vi "Process.vi"(8 "error in (no error)":errorcluster, 10 "Pound in":refnum<class "Pound.lvclass">, 11 "Qbus in":refnum<class "Qbus.lvclass">) -> (0 "error out":errorcluster)   [LabVIEW 2017, in "ServerComm.lvlib"]
doc: "Handles communication between the device and NI InsightCM Server."
uses:
  <vilib>/addons/InsightCM/Devices/Shared/Common/ServerComm/ServerComm.lvlib
  <vilib>/addons/Qbus/Qbus.lvclass
  <vilib>/NI/Software Watchdog/Pound/Pound.lvclass
  <vilib>/addons/InsightCM/Devices/Shared/Common/ServerComm/controls/config.ctl
  <vilib>/addons/InsightCM/MessageBus/TcpApi/controls/TcpMessageReference.ctl
  <vilib>/addons/InsightCM/MessageBus/Base/controls/ConnectionInfo.ctl
  <vilib>/addons/InsightCM/SRP/controls/DVR_data.ctl
  <vilib>/addons/InsightCM/SRP/controls/data.ctl
  <vilib>/addons/InsightCM/Devices/Shared/Common/ServerComm/controls/ConnectedStatusDvr.ctl
  <vilib>/addons/InsightCM/Devices/Shared/Common/ServerComm/controls/ConnectionStatus.ctl
  <vilib>/addons/InsightCM/Devices/Shared/Common/ServerComm/controls/DataSendStatus.ctl
  <vilib>/addons/InsightCM/Devices/Shared/Common/ServerComm/controls/DataSendMode.ctl
  <vilib>/addons/InsightCM/Devices/Shared/Common/ServerComm/controls/ReconnectData.ctl
  <vilib>/addons/InsightCM/Devices/Shared/Common/ServerComm/controls/ProvisioningVersionInfo.ctl
  <vilib>/addons/InsightCM/MessageBus/MessageLibrary/Authentication/controls/AuthSrpVerificationRequestBody.ctl
  <vilib>/addons/InsightCM/Devices/Shared/Common/ServerComm/controls/TimerFunction.ctl
  <vilib>/addons/InsightCM/MessageBus/MessageLibrary/Transceiver/controls/TransAuthorizePortRequestBody.ctl
  <vilib>/addons/InsightCM/MessageBus/MessageLibrary/Device/controls/DeviceInvalidConfigurationBroadcastBody.ctl
  <vilib>/addons/InsightCM/MessageBus/Base/controls/IRoutingSource.ctl
  <vilib>/addons/InsightCM/Devices/Shared/Common/ServerComm/controls/DataSendBody.ctl
  <vilib>/addons/InsightCM/MessageBus/MessageLibrary/Authentication/controls/AuthSrpInitiationRequestBody.ctl
  <vilib>/addons/InsightCM/MessageBus/MessageLibrary/DataStorage/controls/DataStorageOpenEventRequestBody.ctl
  <vilib>/addons/InsightCM/MessageBus/Base/controls/KeyValuePair.ctl
  <vilib>/addons/TraceLogger/TraceLogger.lvlib
  <vilib>/NI/Software Watchdog/Watchdog/Watchdog.lvclass
  <vilib>/addons/InsightCM/SRP/SRP.lvlib
  <vilib>/addons/InsightCM/Utilities/GlobalConfiguration/GlobalConfiguration.lvlib
  <vilib>/addons/InsightCM/Devices/Shared/Common/TracePointSynchronizer/TracePointSynchronizer.lvlib
  <vilib>/addons/InsightCM/Devices/Shared/Common/USBDrive/USBDrive.lvlib
  <vilib>/addons/SystemInfoProcess/SystemInfoProcess.lvlib
  <vilib>/addons/InsightCM/Utilities/PropertyHelpers/PropertyHelpers.lvlib
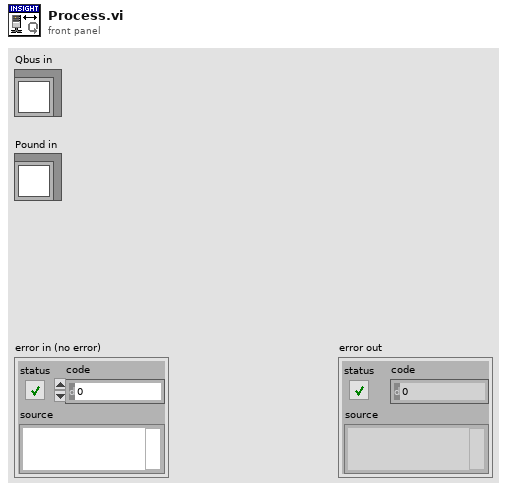
[diagram p1: front panel]
types:
  T1 = typedef "ServerComm.lvlib/config.ctl" = cluster{"tcp":T2, "ConnInfo":T3, "SRP":T4, "connected":T5, "DataSend":T6, "Reconnect":T8, "ProvVersionInfo":T9}
  T2 = typedef "TcpMessageReference.ctl" = refnum<data-value>
  T3 = typedef "ConnectionInfo.ctl" = cluster{"ClientName":string, "TransceiverHost":string, "TransceiverPort":u16, "Password":string}
  T4 = typedef "SRP.lvlib/DVR_data.ctl" = refnum<data-value>
  T5 = typedef "ServerComm.lvlib/ConnectedStatusDvr.ctl" = refnum<data-value>
  T6 = typedef "ServerComm.lvlib/DataSendStatus.ctl" = cluster{"SendFileMode":T7, "data":variant, "InProgress":bool}
  T7 = typedef "ServerComm.lvlib/DataSendMode.ctl" = enum16{"File", "InMemoryFile", "Stream", "StreamFileBlock", "ByteArray", "NoOp", "UnknownData"}
  T8 = typedef "ServerComm.lvlib/ReconnectData.ctl" = cluster{"ReconnectInterval":dbl, "BaseReconnectInterval":dbl, "AuthAttempts":i32, "MaxAttempts":i32}
  T9 = typedef "ServerComm.lvlib/ProvisioningVersionInfo.ctl" = cluster{"ConfigurationVersion":string, "ApplicationVersion":string, "ApplicationType":string}
  T10 = typedef "SectionKeyValues.ctl" = cluster{"Section":string, "KeyValues":T11[]}
  T11 = typedef "KeyValuePair.ctl" = cluster{"Key":string, "Value":string}
  T12 = typedef "ServerComm.lvlib/ConnectionStatus.ctl" = enum16{"Offline", "NotAuthorized", "Online"}
  T13 = typedef "ServerComm.lvlib/TimerFunction.ctl" = enum16{"Start", "Stop", "Reset"}
  T14 = typedef "AuthSrpVerificationRequestBody.ctl" = cluster{"ClientName":string, "ClientHashM":u8[]}
  T15 = typedef "TransAuthorizePortRequestBody.ctl" = cluster{"DeviceName":string, "ConnectionId":string}
  T16 = typedef "DeviceInvalidConfigurationBroadcastBody.ctl" = cluster{"DeviceName":string, "Description":string}
  T17 = typedef "ServerComm.lvlib/DataSendBody.ctl" = cluster{"tcp reference":T2, "SendFileMode":T7, "data":variant, "IRoutingSource":T18, "ReplyTo":string}
  T18 = typedef "IRoutingSource.ctl" = cluster{"CorrelationId":string, "ReplyTo":string}
  T19 = typedef "AuthSrpInitiationRequestBody.ctl" = cluster{"ClientName":string, "PublicKeyA":u8[]}
  T20 = typedef "DataStorageOpenEventRequestBody.ctl" = cluster{"EventId":string, "Properties":T11[]}
  T21 = typedef "Message.ctl" = cluster{"Header":T22, "Body":u8[]}
  T22 = typedef "MessageHeader.ctl" = cluster{"MessageName":string, "Timestamp":i64, "CorrelationId":string, "ContentType":string, "RoutingKey":string, "Properties":T11[]}
  T23 = typedef "AuthSrpInitiationResponseBody.ctl" = cluster{"Salt":u8[], "PublicKeyB":u8[]}
  T24 = typedef "AuthSrpVerificationResponseBody.ctl" = cluster{"ServerHashM":u8[]}
  T25 = typedef "DeviceConnectionInfoUpdateRoutedMessageBody.ctl" = cluster{"IV":u8[], "ConnectionInfo":u8[]}
  T26 = typedef "DeviceConfigurationUpdateRoutedMessageBody.ctl" = cluster{"Config":T27}
  T27 = typedef "DeviceProvisioning.ctl" = cluster{"DeviceModel":T28}
  T28 = typedef "DeviceModel.ctl" = cluster{"Device":T29, "Channels":T38[], "Tags":T39[]}
  T29 = typedef "Device.ctl" = cluster{"Id":string, "Name":string, "DeviceType":string, "HardwareName":string, "IpAddress":string, "HardwareInfo":T11[], "ApplicationType":string, "ApplicationVersion":string, "ConfigurationVersion":string, "State":T30, "Properties":T11[], "DataGroups":T31[], "BurstModeTrigger":T32, "SensorGroups":T35[], "HasSensorGroups":bool, "Endpoints":T36[]}
  T30 = typedef "DeviceState.ctl" = cluster{"Disabled":bool}
  T31 = typedef "DataGroup.ctl" = cluster{"Name":string, "AssetNodeId":string}
  T32 = typedef "BurstModeTrigger.ctl" = cluster{"Trigger":T33, "SampleRate":string, "AcquisitionLength":string}
  T33 = typedef "Trigger.ctl" = cluster{"Type":string, "Expression":string, "Conditions":T34[]}
  T34 = typedef "Condition.ctl" = cluster{"Source":string, "Type":string, "Operator":string, "CompareTo":string, "DwellSeconds":dbl}
  T35 = typedef "DeviceSensorGroup.ctl" = cluster{"EquipId":string, "SensorGroupId":string}
  T36 = typedef "WirelessEndpoint.ctl" = cluster{"SerialNumber":string, "Properties":T11[], "Channels":T37[]}
  T37 = typedef "WirelessChannel.ctl" = cluster{"ChannelNumber":i32, "AssetId":string}
  T38 = typedef "Channel.ctl" = cluster{"Id":string, "DeviceId":string, "ChannelType":string, "HardwareKey":string, "HardwareChannel":string, "DataGroup":string, "Properties":T11[], "AssetNodeId":string}
  T39 = typedef "Tag.ctl" = cluster{"Id":string, "Path":string, "Name":string, "Datatype":string, "Props":T11[], "Keywords":string[]}
  T40 = typedef "DeviceSetNiAuthPasswordRequestBody.ctl" = cluster{"IV":u8[], "Password":u8[]}
  T41 = typedef "ServerComm.lvlib/UpdatePassword.ctl" = cluster{"Device Id":string, "Serial Number":string, "New Password":string}
  T42 = typedef "R2_Device.ctl" = cluster{"Id":string, "Name":string, "DeviceType":string, "HardwareName":string, "IpAddress":string, "HardwareInfo":T11[], "ApplicationType":string, "ApplicationVersion":string, "EquipmentIds":string[], "ConfigurationVersion":string, "State":T30, "Properties":T11[], "DataGroups":T43[], "BurstModeTrigger":T32, "SensorGroups":T35[], "Endpoints":T36[]}
  T43 = typedef "R2_DataGroup.ctl" = cluster{"Name":string, "OperatingStates":T44[], "Properties":T11[], "EquipmentIds":string[], "AssetNodeId":string}
  T44 = typedef "OperatingState.ctl" = cluster{"Name":string, "Properties":T11[], "Triggers":T33[]}
  T45 = typedef "PointValueMap.lvlib/PointMap.ctl" = refnum<data-value>
  T46 = typedef "SystemInfoProcess.lvlib/ImageMetadata.ctl" = cluster{"Title":string, "Description":string, "ID":string, "Version":string}
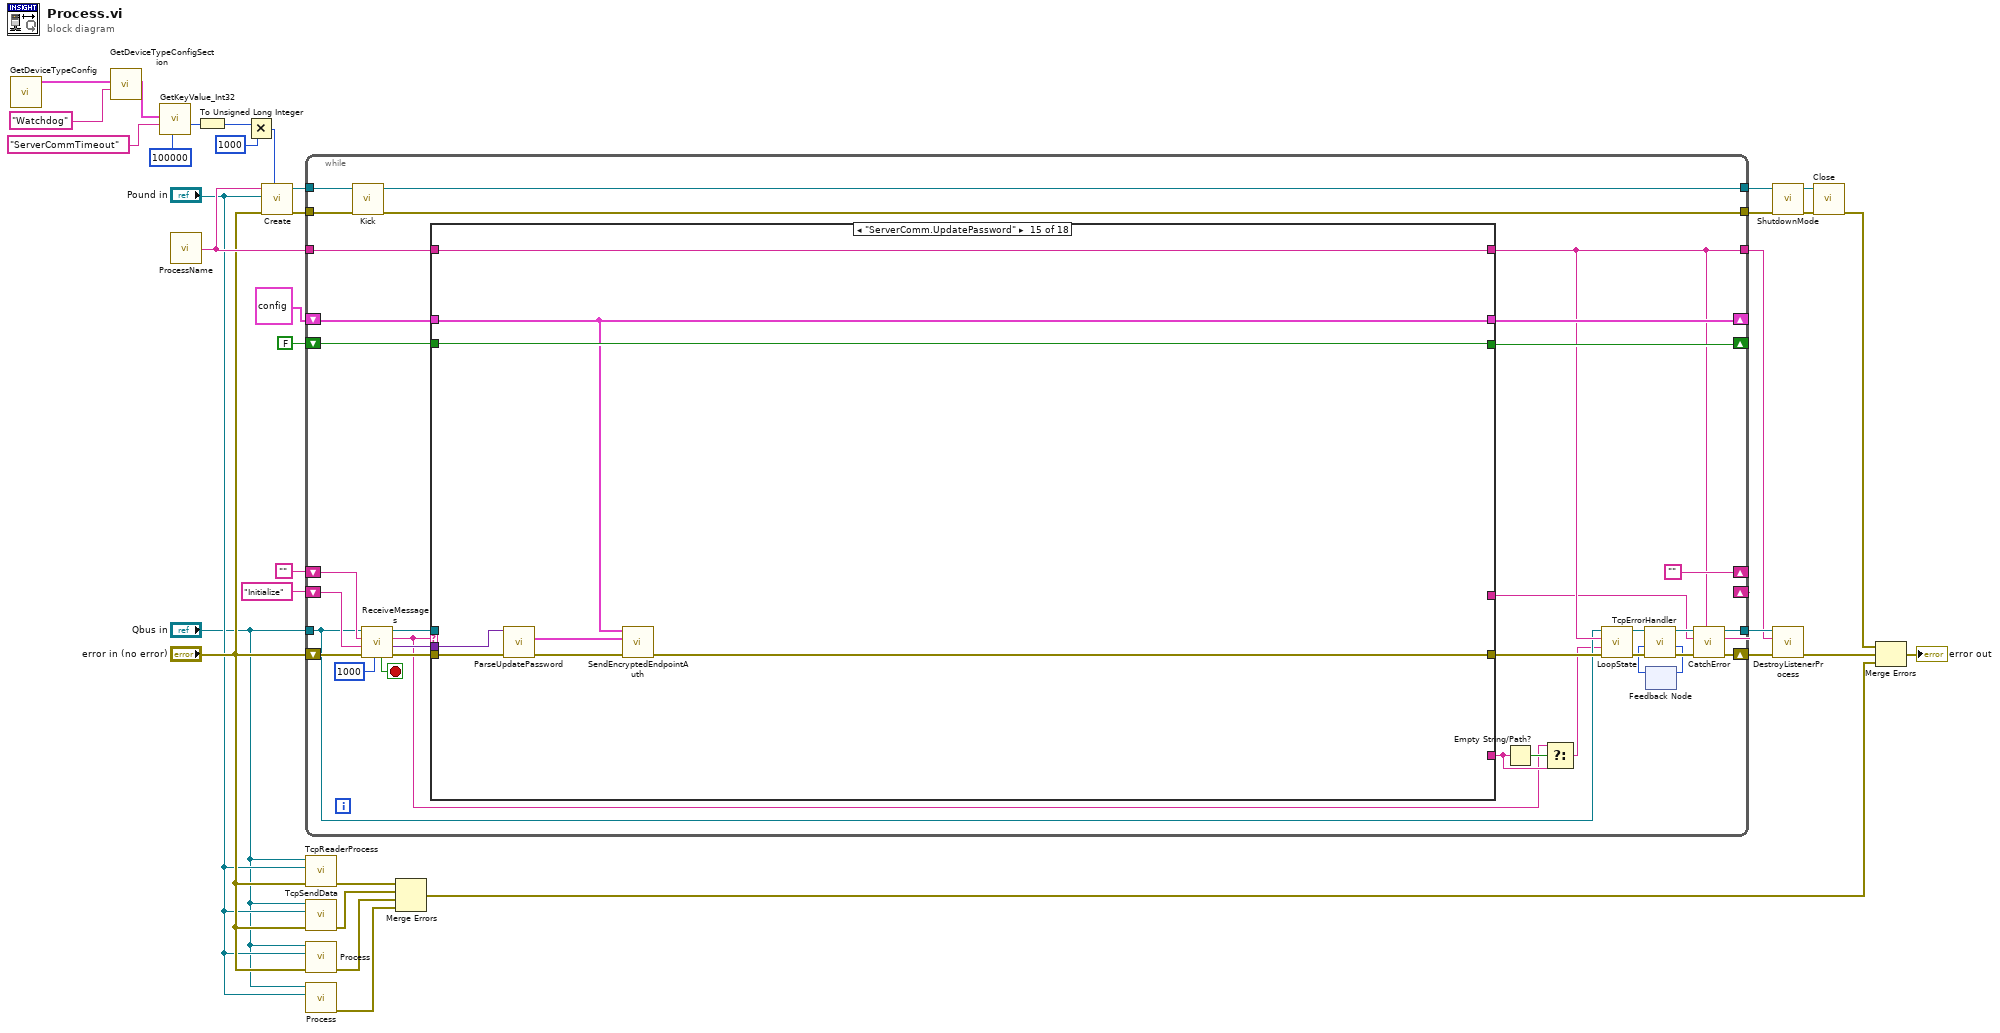
[diagram p0: block diagram]
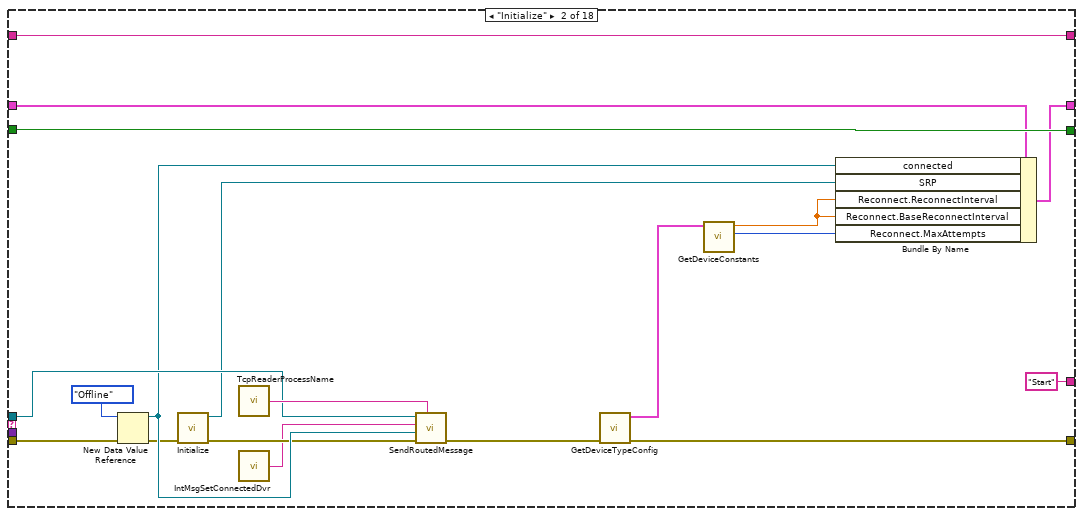
[diagram p3: hidden frame]
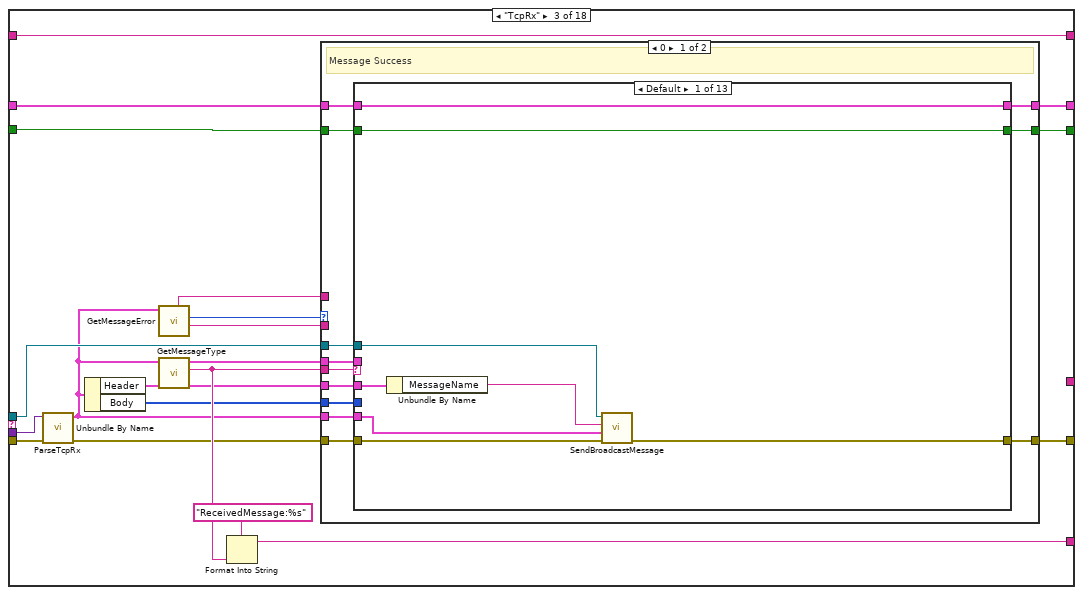
[diagram p4: hidden frame]
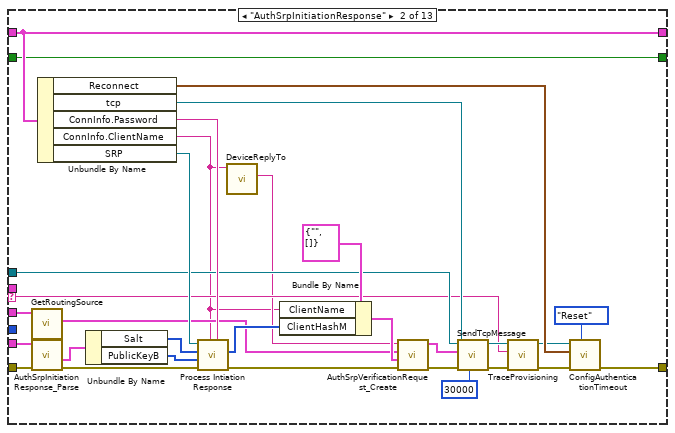
[diagram p5: hidden frame]
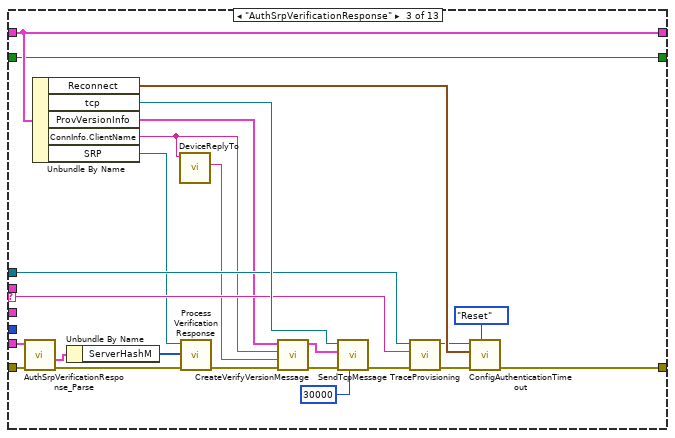
[diagram p6: hidden frame]
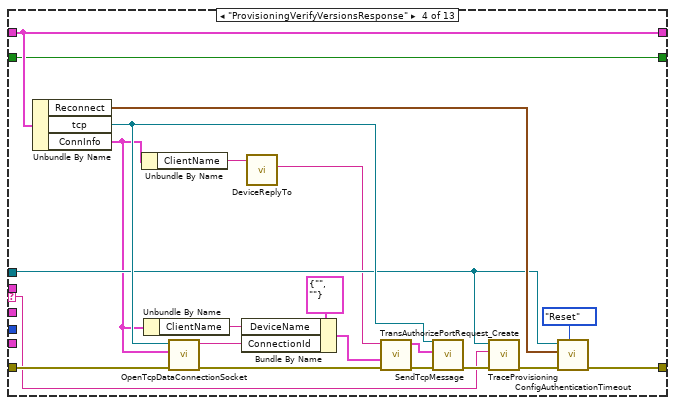
[diagram p7: hidden frame]
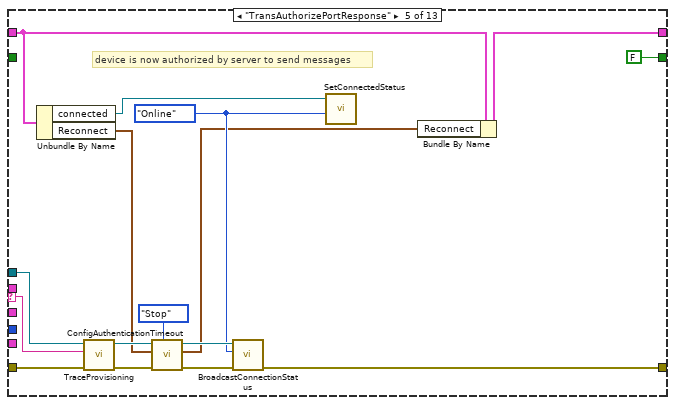
[diagram p8: hidden frame]
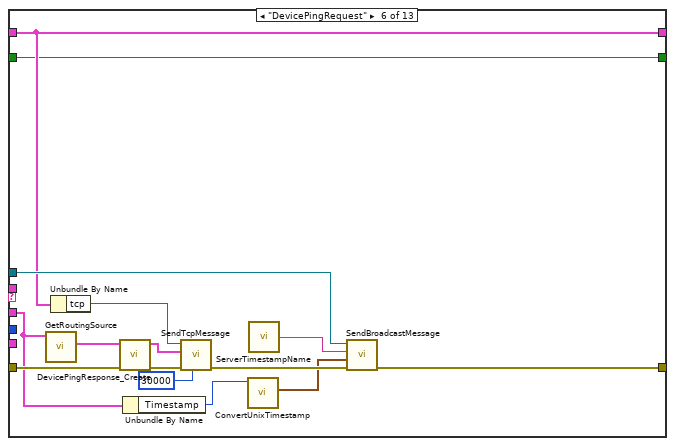
[diagram p9: hidden frame]
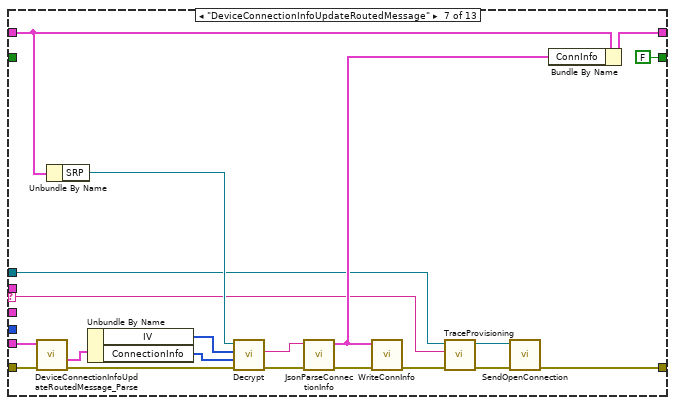
[diagram p10: hidden frame]
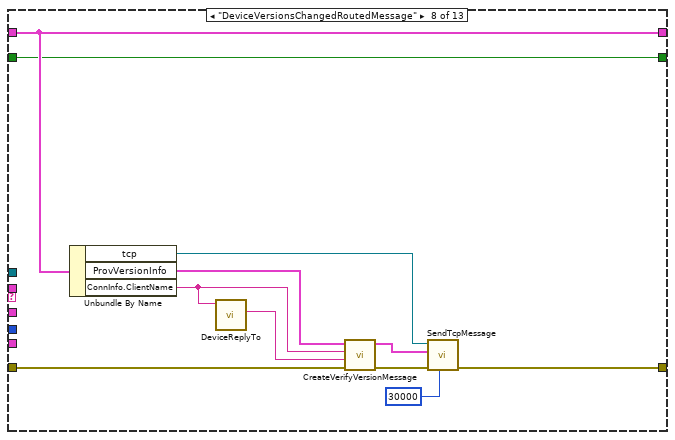
[diagram p11: hidden frame]
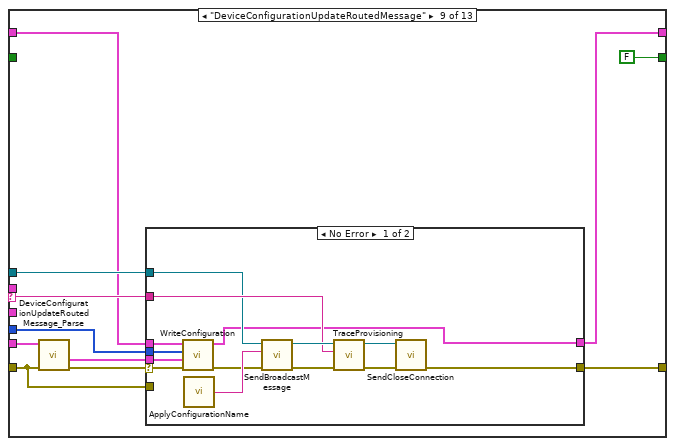
[diagram p12: hidden frame]
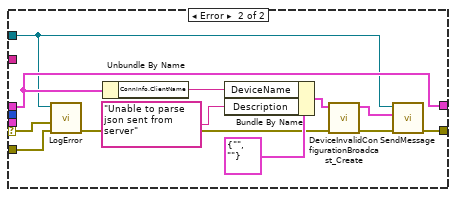
[diagram p13: hidden frame]
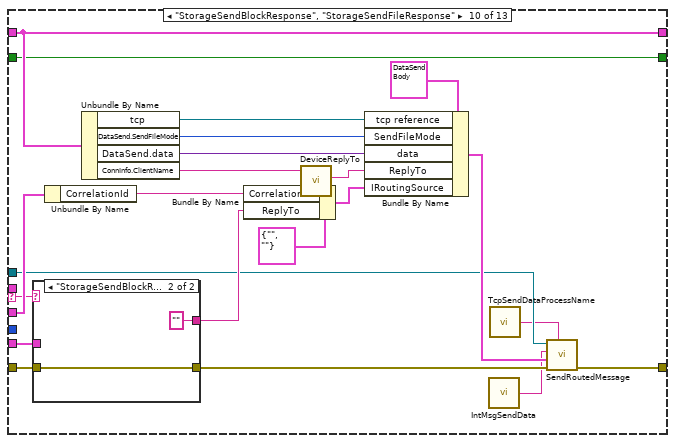
[diagram p14: hidden frame]
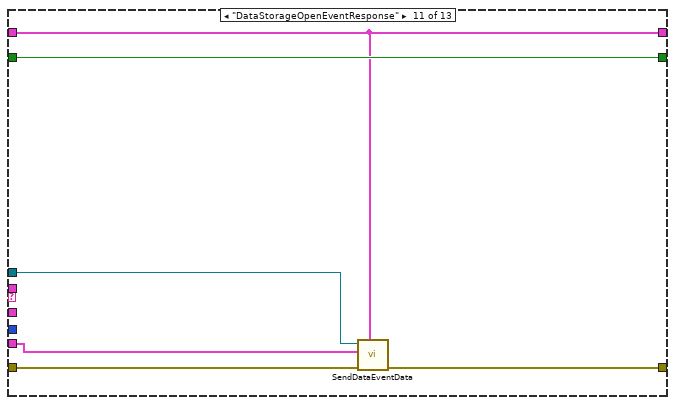
[diagram p16: hidden frame]
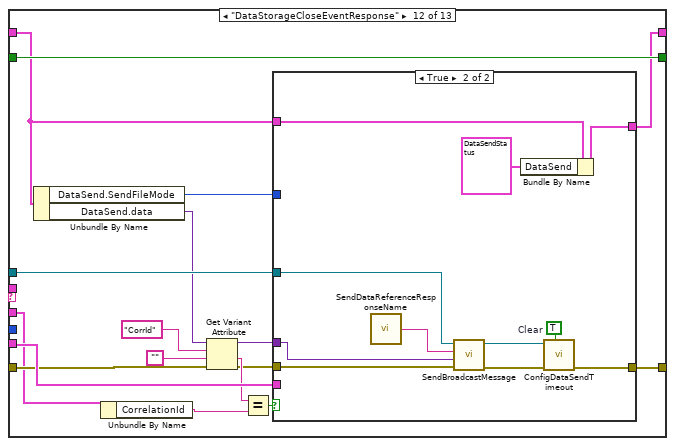
[diagram p17: hidden frame]
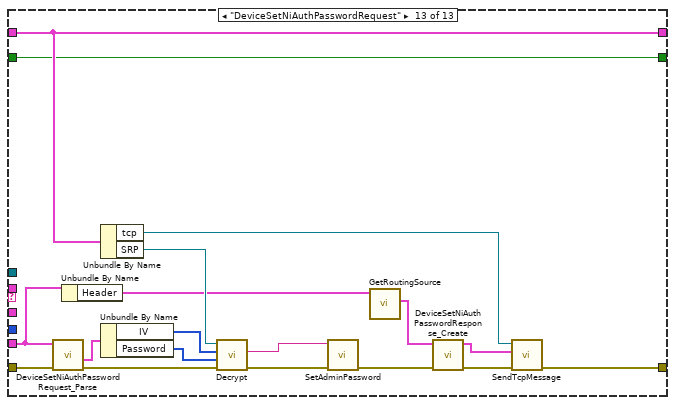
[diagram p19: hidden frame]
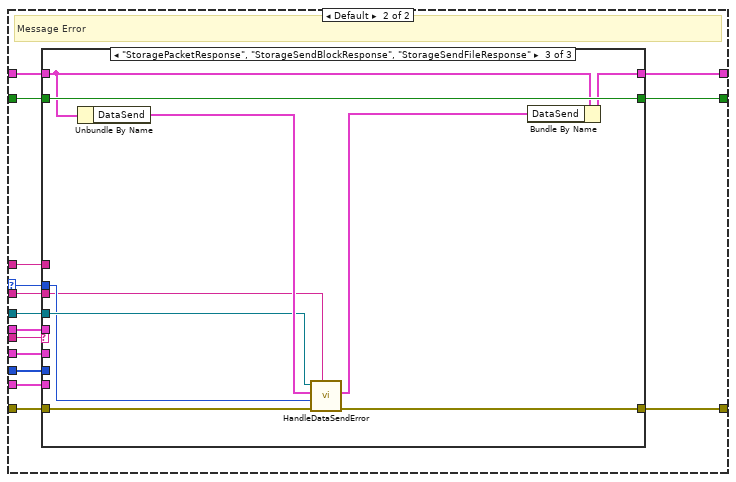
[diagram p20: hidden frame]
diagram:
  n1 = call <vilib>:"GetDeviceTypeConfig.vi"() -> ("key values"=w9:T10[])  [unwired: 9 in, 2 out]
  n2 = call <vilib>:"GetDeviceTypeConfigSection.vi"("key"="Watchdog", "key values"=w9) -> ("key value pairs out"=w7:T11[])  [unwired: 8 in, 1 out]
  n3 = call <vilib>:"GetKeyValue_Int32.vi"("default"=100000 ("Execution Timeout (ms)"), "key"="ServerCommTimeout" ("Tag"), "key value pairs"=w7) -> ("value"=w5:i32)  [unwired: 6 in, 2 out]
  n4 = call <vilib>:"ProcessName.vi"() -> ("process name"=w29:string)  [unwired: 5 in]
  n5 = To Unsigned Long Integer(number=w5) -> (unsigned 32bit integer=w2:u32)
  n6 = Multiply(x=w2, y=u32 1000) -> (x*y=w1:u32)
  n7 = call <vilib>:"Create.vi"("Execution Timeout (ms)"=w1, "error in (no error)"="error in (no error)", "Pound"="Pound in", "Name"=w29) -> ("error out"=w24:errorcluster, "Watchdog"=w28:refnum<data-value>)  [unwired: 6 in]
  n8 = while {
    shift-right: [w65] -> _
    shift-left: FALSE -> [w68]
    shift-right: [""] -> _
    shift-left: "" -> [w67]
    tunnel: "Qbus in" -> [w38]
    tunnel: w29 -> [w37]
    tunnel: [w56] -> w32
    tunnel: [w42] -> w31
    shift-right: [w55] -> _
    shift-left: "Initialize" -> [w61]
    shift-right: [w60] -> _
    shift-left: T1 {"tcp"=refnum, "ConnInfo"={"ClientName"="", "TransceiverHost"="", "TransceiverPort"=0, "Password"=""}, "SRP"=refnum, "connected"=refnum, "DataSend"={"SendFileMode"=enum."File", "data"=variant, "InProgress"=FALSE}, "Reconnect"={"ReconnectInterval"=0.0, "BaseReconnectInterval"=0.0, "AuthAttempts"=0, "MaxAttempts"=10}, "ProvVersionInfo"={"ConfigurationVersion"="", "ApplicationVersion"="", "ApplicationType"=""}} ("state") -> [w35]
    tunnel: w28 -> [w51]
    tunnel: [w50] -> w26
    tunnel: w24 -> [w49]
    tunnel: [w47] -> w23
    shift-right: [w58] -> w33
    shift-left: "error in (no error)" -> [w48]
    stop <- w69 stop-if-true
    n9 = call <vilib>:"Kick.vi"("error in (no error)"=w49, "Watchdog"=w51) -> ("error out"=w47:errorcluster, "Watchdog"=w50:refnum<data-value>)  [unwired: 8 in]
    n10 = call <vilib>:"ReceiveMessages.vi"("timeout(1000)"=1000 ("milliseconds to wait"), "error in (no error)"=w48, "priority action"=w61, "default action"=w67, "Qbus in"=w38) -> ("error out"=w66:errorcluster, "message value"=w62:variant, "action"=w44:string, "Qbus out"=w63:refnum<class "Qbus.lvclass">, "exit"=w69:bool)  [unwired: 2 in]
    n11 = case shown="\"ServerComm.UpdatePassword\"" w44 {
      selector: w44 -> [_ _ _ w437 _ _ _ _ w487 w560 _ _ _ _ _ _ _ _]
      tunnel: w68 -> [w73 w92 w102 _ w454 w469 w478 w484 w486 w565 w576 w584 w597 w628 w672 w691 w701 w713]
      tunnel: w66 -> [w72 w91 w108 w440 w451 w462 w477 w485 w494 w562 w575 w583 w596 w613 w668 w688 w697 w702]
      tunnel: w63 -> [_ w86 w100 w438 w449 w465 w475 _ w491 w557 w569 _ w588 w612 _ w680 w696 w703]
      tunnel: [w72 w79 w105 w435 w450 w466 w476 w485 w490 w553 w568 w582 w589 w626 w670 w678 w698 w709] -> w54
      tunnel: [w73 w92 w101 FALSE w454 w469 w478 w484 TRUE ("OpenConnectionInProgress") w565 w576 w584 w597 w628 w672 w691 w701 w713] -> w65
      tunnel: w62 -> [_ _ w99 _ _ w460 _ _ _ _ w574 w581 w595 w611 w669 _ _ _]
      tunnel: w35 -> [w71 w88 w104 w432 w448 w464 w474 w483 w493 w559 w571 w580 w594 w625 w666 w690 w700 w712]
      tunnel: [w71 w87 w103 w432 w447 w463 w474 w483 w492 w558 w570 w579 w594 w624 w666 w689 w700 w712] -> w60
      tunnel: w37 -> [w70 w89 w98 w430 w445 w455 w471 w482 w488 w552 w566 w577 w587 w615 w671 w677 w699 w704]
      tunnel: [_ _ w106 _ _ _ _ _ _ _ _ _ w585 _ _ _ _ _] -> w45
      tunnel: [w70 w89 w98 w430 w445 w455 w471 w482 w488 w552 w566 w577 w587 w615 w671 w677 w699 w704] -> w42
      tunnel: [_ "Start" ("message name") _ _ _ _ w470 _ _ _ _ _ _ _ _ _ _ _] -> w39
      frame "", Default {
      }
      frame "Initialize" {
        n12 = New Data Value Reference(data value=ConnectionStatus."Offline" ("status"), error in=w91) -> (data value reference=w84:refnum<data-value>, error out=w83:errorcluster)
        n13 = call <vilib>:"Initialize.vi"("error in"=w83) -> ("error out"=w82:errorcluster, "srp"=w81:T4)  [unwired: 9 in]
        n14 = call <vilib>:"TcpReaderProcessName.vi"() -> ("process name"=w90:string)  [unwired: 5 in]
        n15 = call <vilib>:"IntMsgSetConnectedDvr.vi"() -> ("message name"=w80:string)  [unwired: 5 in]
        n16 = call <vilib>:"SendRoutedMessage.vi"("listener process"=w90, "error in (no error)"=w82, "message value"=w84, "message name"=w80, "Qbus in"=w86) -> ("error in (no error)"=w75:errorcluster)  [unwired: 5 in, 1 out]
        n17 = call <vilib>:"GetDeviceTypeConfig.vi"("error in (no error)"=w75) -> ("error out"=w79:errorcluster, "key values"=w78:T10[])  [unwired: 8 in, 1 out]
        n18 = call <vilib>:"GetDeviceConstants.vi"("key values"=w78) -> ("MaxAttempts"=w77:i32, "ReconnectInterval"=w76:dbl)  [unwired: 7 in, 2 out]
        n19 = Bundle By Name(cluster=w88, "connected"=w84, "SRP"=w81, "Reconnect.ReconnectInterval"=w76, "Reconnect.BaseReconnectInterval"=w76, "Reconnect.MaxAttempts"=w77) -> (w87:T1)
      }
      frame "TcpRx" {
        n20 = call <vilib>:"ParseTcpRx.vi"("error in (no error)"=w108, "body"=w99) -> ("error out"=w107:errorcluster, "message"=w96:T21)  [unwired: 8 in]
        n21 = Unbundle By Name(w96) -> ("Header"=w97:T22, "Body"=w109:u8[])
        n22 = call <vilib>:"GetMessageError.vi"("message in"=w96) -> ("error info"=w94:string, "error code"=w95:i32, "error name"=w93:string)  [unwired: 6 in, 2 out]
        n23 = call <vilib>:"GetMessageType.vi"("message in"=w96) -> ("message name"=w111:string, "message out"=w112:T21)  [unwired: 9 in]
        n24 = Format Into String(format string="ReceivedMessage:%s", w111) -> (resulting string=w106:string)  [unwired: 2 in, 1 out]
        n25 = case shown="0" w95 {
          selector: w95 -> [_ w387]
          tunnel: w112 -> [w124 w400]
          tunnel: w111 -> [w123 w399]
          tunnel: w109 -> [w122 w398]
          tunnel: w96 -> [w121 w397]
          tunnel: w107 -> [w120 w396]
          tunnel: [w119 w395] -> w105
          tunnel: w104 -> [w118 w394]
          tunnel: [w117 w388] -> w103
          tunnel: w102 -> [w113 w390]
          tunnel: [w114 w391] -> w101
          tunnel: w100 -> [w116 w393]
          tunnel: w97 -> [w115 w392]
          tunnel: w93 -> [_ w389]
          tunnel: w94 -> [_ w386]
          frame 0 {
            # "Message Success"
            n26 = case shown="Default" w123 {
              selector: w123 -> [_ w140 w174 w193 w220 _ w244 _ w279 w311 _ _ _]
              tunnel: [w131 w146 w179 w197 w212 w227 w242 w266 w277 w315 w336 w352 w371] -> w119
              tunnel: w120 -> [w129 w162 w186 w207 w217 w237 w255 w264 w275 w328 w334 w347 w382]
              tunnel: w115 -> [w126 w137 _ _ _ w232 _ _ _ w327 _ w345 _]
              tunnel: w122 -> [_ _ _ _ _ _ _ _ w272 _ _ _ _]
              tunnel: w118 -> [w132 w145 w178 w199 w216 w229 w243 w269 w271 w317 w332 w339 w380]
              tunnel: [w132 w145 w178 w199 w215 w229 w253 w269 w270 w317 w332 w338 w380] -> w117
              tunnel: w124 -> [_ _ _ _ _ _ _ _ _ _ _ _ _]
              tunnel: w121 -> [w128 w161 w185 _ _ _ w252 _ w280 w326 w333 w351 w376]
              tunnel: w116 -> [w130 w144 w173 w194 w218 w230 w240 _ w273 w313 w337 w353 _]
              tunnel: [w127 w139 w171 w192 FALSE ("OpenConnectionInProgress") w225 FALSE ("OpenConnectionInProgress") w265 FALSE ("OpenConnectionInProgress") w310 w335 w354 w378] -> w114
              tunnel: w113 -> [w127 w139 w171 w192 _ w225 _ w265 _ w310 w335 w354 w378]
              frame Default {
                n27 = Unbundle By Name(w126) -> ("MessageName"=w125:string)
                n28 = call <vilib>:"SendBroadcastMessage.vi"("error in (no error)"=w129, "message value"=w128, "message name"=w125, "Qbus in"=w130) -> ("error in (no error)"=w131:errorcluster)  [unwired: 6 in, 1 out]
              }
              frame "AuthSrpInitiationResponse" {
                n29 = call <vilib>:"GetRoutingSource.vi"("Header in"=w137) -> ("IRoutingSource"=w136:T18)  [unwired: 9 in, 1 out]
                n30 = call <vilib>:"AuthSrpInitiationResponse_Parse.vi"("error in (no error)"=w162, "Message"=w161) -> ("error out"=w158:errorcluster, "Body"=w152:T23)  [unwired: 6 in, 2 out]
                n31 = Unbundle By Name(w145) -> ("Reconnect"=w147:T8, "tcp"=w149:T2, "ConnInfo.Password"=w153:string, "ConnInfo.ClientName"=w133:string, "SRP"=w157:T4)
                n32 = Unbundle By Name(w152) -> ("Salt"=w156:u8[], "PublicKeyB"=w155:u8[])
                n33 = call <vilib>:"Process Intiation Response.vi"("password"=w153, "user name"=w133, "error in (no error)"=w158, "publicKeyB"=w155, "salt"=w156, "srp"=w157) -> ("error out"=w154:errorcluster, "clientHash"=w159:u8[])  [unwired: 3 in, 1 out]
                n34 = call <vilib>:"DeviceReplyTo.vi"("Device"=w133) -> ("ReplyTo"=w134:string)  [unwired: 10 in]
                n35 = Bundle By Name(cluster=T14 {"ClientName"="", "ClientHashM"=[]} ("Body"), "ClientName"=w133, "ClientHashM"=w159) -> (w138:T14)
                n36 = call <vilib>:"AuthSrpVerificationRequest_Create.vi"("error in (no error)"=w154, "AuthSrpVerificationRequest"=w138, "IRoutingSource"=w136, "ReplyTo"=w134) -> ("error out"=w151:errorcluster, "Message"=w148:T21)  [unwired: 6 in]
                n37 = call <vilib>:"SendTcpMessage.vi"("timeout (5 sec)"=30000, "error in (no error)"=w151, "message"=w148, "connection ID in"=w149) -> ("error out"=w142:errorcluster)  [unwired: 5 in, 2 out]
                n38 = call <vilib>:"TraceProvisioning.vi"("error in (no error)"=w142, "message name"=w140, "Qbus in"=w144) -> ("error out"=w141:errorcluster, "Qbus out"=w143:refnum<class "Qbus.lvclass">)  [unwired: 7 in]
                n39 = call <vilib>:"ConfigAuthenticationTimeout.vi"("timer function"=TimerFunction."Reset" ("Timer function"), "error in (no error)"=w141, "reconnect in"=w147, "Qbus in"=w143) -> ("error out"=w146:errorcluster)  [unwired: 5 in, 2 out]
              }
              frame "AuthSrpVerificationResponse" {
                n40 = call <vilib>:"AuthSrpVerificationResponse_Parse.vi"("error in (no error)"=w186, "Message"=w185) -> ("error out"=w184:errorcluster, "Body"=w180:T24)  [unwired: 6 in, 2 out]
                n41 = Unbundle By Name(w178) -> ("Reconnect"=w177:T8, "tcp"=w181:T2, "ProvVersionInfo"=w166:T9, "ConnInfo.ClientName"=w163:string, "SRP"=w167:T4)
                n42 = Unbundle By Name(w180) -> ("ServerHashM"=w183:u8[])
                n43 = call <vilib>:"DeviceReplyTo.vi"("Device"=w163) -> ("ReplyTo"=w164:string)  [unwired: 10 in]
                n44 = call <vilib>:"Process Verification Response.vi"("error in"=w184, "serverHash"=w183, "srp"=w167) -> ("error out"=w169:errorcluster)  [unwired: 7 in, 1 out]
                n45 = call <vilib>:"CreateVerifyVersionMessage.vi"("error in (no error)"=w169, "reply to"=w164, "device name"=w163, "prov version info"=w166) -> ("error out"=w168:errorcluster, "message"=w170:T21)  [unwired: 6 in]
                n46 = call <vilib>:"SendTcpMessage.vi"("timeout (5 sec)"=30000, "error in (no error)"=w168, "message"=w170, "connection ID in"=w181) -> ("error out"=w176:errorcluster)  [unwired: 5 in, 2 out]
                n47 = call <vilib>:"TraceProvisioning.vi"("error in (no error)"=w176, "message name"=w174, "Qbus in"=w173) -> ("error out"=w175:errorcluster, "Qbus out"=w172:refnum<class "Qbus.lvclass">)  [unwired: 7 in]
                n48 = call <vilib>:"ConfigAuthenticationTimeout.vi"("timer function"=TimerFunction."Reset" ("Timer function"), "error in (no error)"=w175, "reconnect in"=w177, "Qbus in"=w172) -> ("error out"=w179:errorcluster)  [unwired: 5 in, 2 out]
              }
              frame "ProvisioningVerifyVersionsResponse" {
                n49 = Unbundle By Name(w199) -> ("Reconnect"=w198:T8, "tcp"=w202:T2, "ConnInfo"=w188:T3)
                n50 = Unbundle By Name(w188) -> ("ClientName"=w187:string)
                n51 = Unbundle By Name(w188) -> ("ClientName"=w191:string)
                n52 = call <vilib>:"OpenTcpDataConnectionSocket.vi"("error in"=w207, "ConnInfo"=w188, "tcp"=w202) -> ("error out"=w204:errorcluster, "ConnectionId"=w205:string)  [unwired: 7 in]
                n53 = Bundle By Name(cluster=T15 {"DeviceName"="", "ConnectionId"=""} ("Body"), "DeviceName"=w191, "ConnectionId"=w205) -> (w201:T15)
                n54 = call <vilib>:"DeviceReplyTo.vi"("Device"=w187) -> ("ReplyTo"=w189:string)  [unwired: 10 in]
                n55 = call <vilib>:"TransAuthorizePortRequest_Create.vi"("error in (no error)"=w204, "TransAuthorizePortRequest"=w201, "ReplyTo"=w189) -> ("error out"=w200:errorcluster, "Message"=w203:T21)  [unwired: 7 in]
                n56 = call <vilib>:"SendTcpMessage.vi"("error in (no error)"=w200, "message"=w203, "connection ID in"=w202) -> ("error out"=w196:errorcluster)  [unwired: 6 in, 2 out]
                n57 = call <vilib>:"TraceProvisioning.vi"("error in (no error)"=w196, "message name"=w193, "Qbus in"=w194) -> ("error out"=w195:errorcluster)  [unwired: 7 in, 1 out]
                n58 = call <vilib>:"ConfigAuthenticationTimeout.vi"("timer function"=TimerFunction."Reset" ("Timer function"), "error in (no error)"=w195, "reconnect in"=w198, "Qbus in"=w194) -> ("error out"=w197:errorcluster)  [unwired: 5 in, 2 out]
              }
              frame "TransAuthorizePortResponse" {
                w211 = ConnectionStatus."Online" ("status")
                # "device is now authorized by server to send messages"
                n59 = Unbundle By Name(w216) -> ("connected"=w223:T5, "Reconnect"=w210:T8)
                n60 = call <vilib>:"TraceProvisioning.vi"("error in (no error)"=w217, "message name"=w220, "Qbus in"=w218) -> ("error out"=w221:errorcluster, "Qbus out"=w222:refnum<class "Qbus.lvclass">)  [unwired: 7 in]
                n61 = call <vilib>:"ConfigAuthenticationTimeout.vi"("timer function"=TimerFunction."Stop" ("Timer function"), "error in (no error)"=w221, "reconnect in"=w210, "Qbus in"=w222) -> ("error out"=w213:errorcluster, "reconnect out"=w209:T8, "Qbus out"=w214:refnum<class "Qbus.lvclass">)  [unwired: 5 in]
                n62 = call <vilib>:"BroadcastConnectionStatus.vi"("error in (no error)"=w213, "status"=w211, "Qbus in"=w214) -> ("error out"=w212:errorcluster)  [unwired: 7 in, 1 out]
                n63 = call <vilib>:"SetConnectedStatus.vi"("status"=w211, "dvrConnected"=w223) -> ()  [unwired: 5 in, 1 out]
                n64 = Bundle By Name(cluster=w216, "Reconnect"=w209) -> (w215:T1)
              }
              frame "DevicePingRequest" {
                n65 = call <vilib>:"GetRoutingSource.vi"("Header in"=w232) -> ("IRoutingSource"=w231:T18)  [unwired: 9 in, 1 out]
                n66 = Unbundle By Name(w229) -> ("tcp"=w234:T2)
                n67 = call <vilib>:"DevicePingResponse_Create.vi"("error in (no error)"=w237, "IRoutingSource"=w231) -> ("error out"=w236:errorcluster, "Message"=w233:T21)  [unwired: 8 in]
                n68 = Unbundle By Name(w232) -> ("Timestamp"=w238:i64)
                n69 = call <vilib>:"SendTcpMessage.vi"("timeout (5 sec)"=30000, "error in (no error)"=w236, "message"=w233, "connection ID in"=w234) -> ("error out"=w228:errorcluster)  [unwired: 5 in, 2 out]
                n70 = call <vilib>:"ConvertUnixTimestamp.vi"("Timestamp in"=w238) -> ("Time Stamp out"=w226:timestamp)  [unwired: 10 in]
                n71 = call <vilib>:"ServerTimestampName.vi"() -> ("message name"=w224:string)  [unwired: 5 in]
                n72 = call <vilib>:"SendBroadcastMessage.vi"("error in (no error)"=w228, "message value"=w226, "message name"=w224, "Qbus in"=w230) -> ("error in (no error)"=w227:errorcluster)  [unwired: 6 in, 1 out]
              }
              frame "DeviceConnectionInfoUpdateRoutedMessage" {
                n73 = call <vilib>:"DeviceConnectionInfoUpdateRoutedMessage_Parse.vi"("error in (no error)"=w255, "Message"=w252) -> ("error out"=w258:errorcluster, "Body"=w251:T25)  [unwired: 6 in, 2 out]
                n74 = Unbundle By Name(w243) -> ("SRP"=w254:T4)
                n75 = Unbundle By Name(w251) -> ("IV"=w257:u8[], "ConnectionInfo"=w256:u8[])
                n76 = call <vilib>:"Decrypt.vi"("error in (no error)"=w258, "Configuration"=w256, "IV"=w257, "srp"=w254) -> ("error out"=w249:errorcluster, "output"=w250:string)  [unwired: 5 in, 1 out]
                n77 = call <vilib>:"JsonParseConnectionInfo.vi"("error in (no error)"=w249, "JSON string"=w250) -> ("error out"=w248:errorcluster, "connection info"=w247:T3)  [unwired: 8 in]
                n78 = call <vilib>:"WriteConnInfo.vi"("error in (no error)"=w248, "connection info"=w247) -> ("error out"=w246:errorcluster)  [unwired: 9 in]
                n79 = call <vilib>:"TraceProvisioning.vi"("error in (no error)"=w246, "message name"=w244, "Qbus in"=w240) -> ("error out"=w245:errorcluster, "Qbus out"=w239:refnum<class "Qbus.lvclass">)  [unwired: 7 in]
                n80 = call <vilib>:"SendOpenConnection.vi"("error in (no error)"=w245, "Qbus in"=w239) -> ("error out"=w242:errorcluster)  [unwired: 8 in, 1 out]
                n81 = Bundle By Name(cluster=w243, "ConnInfo"=w247) -> (w253:T1)
              }
              frame "DeviceVersionsChangedRoutedMessage" {
                n82 = Unbundle By Name(w269) -> ("tcp"=w267:T2, "ProvVersionInfo"=w262:T9, "ConnInfo.ClientName"=w259:string)
                n83 = call <vilib>:"DeviceReplyTo.vi"("Device"=w259) -> ("ReplyTo"=w260:string)  [unwired: 10 in]
                n84 = call <vilib>:"CreateVerifyVersionMessage.vi"("error in (no error)"=w264, "reply to"=w260, "device name"=w259, "prov version info"=w262) -> ("error out"=w263:errorcluster, "message"=w261:T21)  [unwired: 6 in]
                n85 = call <vilib>:"SendTcpMessage.vi"("timeout (5 sec)"=30000, "error in (no error)"=w263, "message"=w261, "connection ID in"=w267) -> ("error out"=w266:errorcluster)  [unwired: 5 in, 2 out]
              }
              frame "DeviceConfigurationUpdateRoutedMessage" {
                n86 = call <vilib>:"DeviceConfigurationUpdateRoutedMessage_Parse.vi"("error in (no error)"=w275, "Message"=w280) -> ("error out"=w276:errorcluster, "Body"=w274:T26)  [unwired: 6 in, 2 out]
                n87 = case shown="No Error" w276 {
                  selector: w276 -> [w287 w297]
                  tunnel: w279 -> [w292 _]
                  tunnel: [w290 w299] -> w277
                  tunnel: w275 -> [_ w296]
                  tunnel: w274 -> [w281 _]
                  tunnel: w271 -> [w286 w300]
                  tunnel: w273 -> [w284 w298]
                  tunnel: [w283 w300] -> w270
                  tunnel: w272 -> [w282 _]
                  frame No Error {
                    n88 = call <vilib>:"WriteConfiguration.vi"("error in (no error)"=w287, "msg body"=w281, "body"=w282, "config"=w286) -> ("error out"=w285:errorcluster, "config out"=w283:T1)  [unwired: 6 in]
                    n89 = call <vilib>:"ApplyConfigurationName.vi"() -> ("message name"=w288:string)  [unwired: 5 in]
                    n90 = call <vilib>:"SendBroadcastMessage.vi"("error in (no error)"=w285, "message name"=w288, "Qbus in"=w284) -> ("error in (no error)"=w293:errorcluster, "Qbus out"=w294:refnum<class "Qbus.lvclass">)  [unwired: 7 in]
                    n91 = call <vilib>:"TraceProvisioning.vi"("error in (no error)"=w293, "message name"=w292, "Qbus in"=w294) -> ("error out"=w291:errorcluster, "Qbus out"=w289:refnum<class "Qbus.lvclass">)  [unwired: 7 in]
                    n92 = call <vilib>:"SendCloseConnection.vi"("error in (no error)"=w291, "Qbus in"=w289) -> ("error out"=w290:errorcluster)  [unwired: 8 in, 1 out]
                  }
                  frame Error {
                    n93 = call <vilib>:"LogError.vi"("error in (no error)"=w296, "error"=w297, "qbus in"=w298) -> ("error out"=w295:errorcluster)  [unwired: 7 in, 1 out]
                    n94 = Unbundle By Name(w300) -> ("ConnInfo.ClientName"=w305:string)
                    n95 = Bundle By Name(cluster=T16 {"DeviceName"="", "Description"=""} ("DeviceInvalidConfigurationBroadcast"), "DeviceName"=w305, "Description"="Unable to parse json sent from server") -> (w306:T16)
                    n96 = call <vilib>:"DeviceInvalidConfigurationBroadcast_Create.vi"("error in (no error)"=w295, "DeviceInvalidConfigurationBroadcast"=w306) -> ("error out"=w303:errorcluster, "Message"=w302:T21)  [unwired: 8 in]
                    n97 = call <vilib>:"SendMessage.vi"("error in (no error)"=w303, "message"=w302, "Qbus in"=w298) -> ("error out"=w299:errorcluster)  [unwired: 7 in, 1 out]
                  }
                }
              }
              frame "StorageSendBlockResponse", "StorageSendFileResponse" {
                n98 = case shown="\"StorageSendBlockResponse\"" w311 {
                  tunnel: w328 -> [w329 w330]
                  tunnel: w326 -> [_ _]
                  tunnel: [_ "" ("StorageInstance")] -> w323
                  tunnel: [w329 w330] -> w316
                  frame "StorageSendFileResponse", Default {
                  }
                  frame "StorageSendBlockResponse" {
                  }
                }
                n99 = Unbundle By Name(w327) -> ("CorrelationId"=w324:string)
                n100 = Unbundle By Name(w317) -> ("tcp"=w320:T2, "DataSend.SendFileMode"=w319:T7, "DataSend.data"=w318:variant, "ConnInfo.ClientName"=w307:string)
                n101 = Bundle By Name(cluster=T18 {"CorrelationId"="", "ReplyTo"=""} ("IRoutingSource"), "CorrelationId"=w324, "ReplyTo"=w323) -> (w321:T18)
                n102 = call <vilib>:"DeviceReplyTo.vi"("Device"=w307) -> ("ReplyTo"=w308:string)  [unwired: 10 in]
                n103 = Bundle By Name(cluster=T17 {"tcp reference"=refnum, "SendFileMode"=enum."File", "data"=variant, "IRoutingSource"={"CorrelationId"="", "ReplyTo"=""}, "ReplyTo"=""} ("DataSend"), "tcp reference"=w320, "SendFileMode"=w319, "data"=w318, "ReplyTo"=w308, "IRoutingSource"=w321) -> (w314:T17)
                n104 = call <vilib>:"IntMsgSendData.vi"() -> ("message name"=w309:string)  [unwired: 5 in]
                n105 = call <vilib>:"TcpSendDataProcessName.vi"() -> ("process name"=w312:string)  [unwired: 5 in]
                n106 = call <vilib>:"SendRoutedMessage.vi"("listener process"=w312, "error in (no error)"=w316, "message value"=w314, "message name"=w309, "Qbus in"=w313) -> ("error in (no error)"=w315:errorcluster)  [unwired: 5 in, 1 out]
              }
              frame "DataStorageOpenEventResponse" {
                n107 = call <vilib>:"SendDataEventData.vi"("state in"=w332, "error in (no error)"=w334, "message"=w333, "Qbus in"=w337) -> ("error out"=w336:errorcluster)  [unwired: 7 in]
              }
              frame "DataStorageCloseEventResponse" {
                n108 = Unbundle By Name(w339) -> ("DataSend.SendFileMode"=w342:T7, "DataSend.data"=w341:variant)
                n109 = Unbundle By Name(w345) -> ("CorrelationId"=w344:string)
                n110 = Get Variant Attribute(Variant=w341, name="CorrId", default value (empty Variant)="", error in=w347) -> (duplicate Variant=w340:variant, value=w348:string, error out=w346:errorcluster)  [unwired: 1 out]
                n111 = Equal?(x=w348, y=w344) -> (x = y?=w343:bool)
                n112 = case shown="True" w343 {
                  tunnel: w353 -> [_ w364]
                  tunnel: [w356 w360] -> w352
                  tunnel: w351 -> [_ _]
                  tunnel: w346 -> [w356 w362]
                  tunnel: w342 -> [_ _]
                  tunnel: w340 -> [_ w365]
                  tunnel: w339 -> [w355 w358]
                  tunnel: [w355 w357] -> w338
                  frame False {
                  }
                  frame True {
                    w367 = TRUE  # Clear
                    n113 = call <vilib>:"SendDataReferenceResponseName.vi"() -> ("message name"=w366:string)  [unwired: 5 in]
                    n114 = call <vilib>:"SendBroadcastMessage.vi"("error in (no error)"=w362, "message value"=w365, "message name"=w366, "Qbus in"=w364) -> ("error in (no error)"=w361:errorcluster, "Qbus out"=w363:refnum<class "Qbus.lvclass">)  [unwired: 6 in]
                    n115 = Bundle By Name(cluster=w358, "DataSend"=T6 {"SendFileMode"=enum."File", "data"=variant, "InProgress"=FALSE}) -> (w357:T1)
                    n116 = call <vilib>:"ConfigDataSendTimeout.vi"("clear"=w367, "error in (no error)"=w361, "Qbus in"=w363) -> ("error out"=w360:errorcluster)  [unwired: 7 in, 1 out]
                  }
                }
              }
              frame "DeviceSetNiAuthPasswordRequest" {
                n117 = call <vilib>:"DeviceSetNiAuthPasswordRequest_Parse.vi"("error in (no error)"=w382, "Message"=w376) -> ("error out"=w381:errorcluster, "Body"=w379:T40)  [unwired: 6 in, 2 out]
                n118 = Unbundle By Name(w376) -> ("Header"=w368:T22)
                n119 = Unbundle By Name(w380) -> ("tcp"=w370:T2, "SRP"=w383:T4)
                n120 = Unbundle By Name(w379) -> ("IV"=w385:u8[], "Password"=w384:u8[])
                n121 = call <vilib>:"Decrypt.vi"("error in (no error)"=w381, "Configuration"=w384, "IV"=w385, "srp"=w383) -> ("error out"=w375:errorcluster, "output"=w377:string)  [unwired: 5 in, 1 out]
                n122 = call <vilib>:"SetAdminPassword.vi"("error in"=w375, "New Password"=w377) -> ("error out"=w374:errorcluster)  [unwired: 9 in]
                n123 = call <vilib>:"GetRoutingSource.vi"("Header in"=w368) -> ("IRoutingSource"=w369:T18)  [unwired: 9 in, 1 out]
                n124 = call <vilib>:"DeviceSetNiAuthPasswordResponse_Create.vi"("error in (no error)"=w374, "IRoutingSource"=w369) -> ("error out"=w372:errorcluster, "Message"=w373:T21)  [unwired: 8 in]
                n125 = call <vilib>:"SendTcpMessage.vi"("error in (no error)"=w372, "message"=w373, "connection ID in"=w370) -> ("error out"=w371:errorcluster)  [unwired: 6 in, 2 out]
              }
            }
          }
          frame Default {
            # "Message Error"
            n126 = case shown="\"StoragePacketResponse\", \"StorageSendBlockResponse\", \"StorageSendFileResponse\"" w399 {
              selector: w399 -> [_ w418 _]
              tunnel: [w407 w413 w425] -> w395
              tunnel: w396 -> [w405 w419 w426]
              tunnel: w392 -> [w402 _ _]
              tunnel: w398 -> [_ _ _]
              tunnel: w394 -> [w408 w411 w427]
              tunnel: [w408 w411 w428] -> w388
              tunnel: w400 -> [_ _ _]
              tunnel: w397 -> [w404 _ _]
              tunnel: w393 -> [w406 w416 w422]
              tunnel: [w403 FALSE w429] -> w391
              tunnel: w390 -> [w403 _ w429]
              tunnel: w389 -> [_ w417 _]
              tunnel: w387 -> [_ _ w421]
              tunnel: w386 -> [_ _ w420]
              frame Default {
                n127 = Unbundle By Name(w402) -> ("MessageName"=w401:string)
                n128 = call <vilib>:"SendBroadcastMessage.vi"("error in (no error)"=w405, "message value"=w404, "message name"=w401, "Qbus in"=w406) -> ("error in (no error)"=w407:errorcluster)  [unwired: 6 in, 1 out]
              }
              frame "AuthSrpInitiationResponse", "AuthSrpVerificationResponse", "ProvisioningVerifyVersionsResponse", "TransAuthorizePortResponse" {
                n129 = Unbundle By Name(w411) -> ("tcp"=w415:T2, "connected"=w414:T5)
                n130 = call <vilib>:"TraceProvisioning.vi"("error in (no error)"=w419, "addional info"=w417, "message name"=w418, "Qbus in"=w416) -> ("error out"=w409:errorcluster, "Qbus out"=w410:refnum<class "Qbus.lvclass">)  [unwired: 6 in]
                n131 = call <vilib>:"CloseConnectionInternal.vi"("error in (no error)"=w409, "Qbus in"=w410, "connected"=w414, "tcp reference"=w415) -> ("error out"=w413:errorcluster)  [unwired: 7 in]
              }
              frame "StoragePacketResponse", "StorageSendBlockResponse", "StorageSendFileResponse" {
                n132 = Unbundle By Name(w427) -> ("DataSend"=w424:T6)
                n133 = call <vilib>:"HandleDataSendError.vi"("error info"=w420, "error in (no error)"=w426, "error code"=w421, "data send in"=w424, "Qbus in"=w422) -> ("error out"=w425:errorcluster, "data send out"=w423:T6)  [unwired: 4 in, 1 out]
                n134 = Bundle By Name(cluster=w427, "DataSend"=w423) -> (w428:T1)
              }
            }
          }
        }
      }
      frame "AuthenticationTimeout" {
        n135 = call <vilib>:"TraceProvisioning.vi"("error in (no error)"=w440, "message name"=w437, "Qbus in"=w438) -> ("error out"=w433:errorcluster, "Qbus out"=w434:refnum<class "Qbus.lvclass">)  [unwired: 7 in]
        n136 = Unbundle By Name(w432) -> ("Reconnect.ReconnectInterval"=w431:dbl)
        n137 = Greater Than 0?(x=w431) -> (x > 0?=w436:bool)
        n138 = case shown="True" w436 {
          tunnel: w434 -> [_ w444]
          tunnel: w433 -> [w441 w443]
          tunnel: [w441 w442] -> w435
          frame False {
          }
          frame True {
            n139 = call <vilib>:"SendOpenConnection.vi"("error in (no error)"=w443, "Qbus in"=w444) -> ("error out"=w442:errorcluster)  [unwired: 8 in, 1 out]
          }
        }
      }
      frame "SendDataTimeout" {
        w446 = -386728  # TimeoutSendingData
        n140 = Unbundle By Name(w448) -> ("DataSend"=w453:T6)
        n141 = call <vilib>:"HandleDataSendError.vi"("error in (no error)"=w451, "error code"=w446, "data send in"=w453, "Qbus in"=w449) -> ("error out"=w450:errorcluster, "data send out"=w452:T6)  [unwired: 5 in, 1 out]
        n142 = Bundle By Name(cluster=w448, "DataSend"=w452) -> (w447:T1)
      }
      frame "FileError" {
        n143 = Unbundle By Name(w464) -> ("DataSend"=w468:T6)
        n144 = Variant To Data(error in=w462, type=errorcluster {"status"=FALSE, "code"=0, "source"=""} ("error out"), Variant=w460) -> (data=w458:errorcluster, error out=w461:errorcluster)
        n145 = Unbundle By Name(w458) -> ("source"=w456:string, "code"=w457:i32)
        n146 = call <vilib>:"HandleDataSendError.vi"("error info"=w456, "error in (no error)"=w461, "error code"=w457, "data send in"=w468, "Qbus in"=w465) -> ("error out"=w466:errorcluster, "data send out"=w467:T6)  [unwired: 4 in, 1 out]
        n147 = Bundle By Name(cluster=w464, "DataSend"=w467) -> (w463:T1)
      }
      frame "TcpError" {
        n148 = Unbundle By Name(w474) -> ("connected"=w473:T5)
        n149 = call <vilib>:"GetConnectedStatus.vi"("dvr connected"=w473) -> ("status"=w472:T12)  [unwired: 5 in, 1 out]
        n150 = case shown="\"NotAuthorized\", \"Online\"" w472 {
          tunnel: w477 -> [w479 w481]
          tunnel: [w479 w481] -> w476
          tunnel: w475 -> [_ _]
          tunnel: [_ w480] -> w470
          frame "Offline", Default {
          }
          frame "NotAuthorized", "Online" {
            n151 = call <vilib>:"MsgOpenConnection.vi"() -> ("message name"=w480:string)  [unwired: 5 in]
          }
        }
      }
      frame "<----------- From Outside Process ----------->" {
      }
      frame "ServerComm.OpenConnection" {
        n152 = case shown="False" w486 {
          tunnel: w494 -> [w524 w549]
          tunnel: w487 -> [w501 _]
          tunnel: w493 -> [w502 w550]
          tunnel: [w522 w550] -> w492
          tunnel: w491 -> [w519 _]
          tunnel: [w506 w549] -> w490
          frame False {
            w500 = 10000 ("timeout ms (25000)")
            n153 = Unbundle By Name(w502) -> ("Reconnect"=w513:T8, "ConnInfo.ClientName"=w504:string, "SRP"=w521:T4, "ConnInfo.TransceiverHost"=w528:string, "ConnInfo.TransceiverPort"=w527:u16, "tcp"=w529:T2, "connected"=w525:T5)
            n154 = call <vilib>:"TraceProvisioning.vi"("error in (no error)"=w524, "message name"=w501, "Qbus in"=w519) -> ("error out"=w499:errorcluster, "Qbus out"=w498:refnum<class "Qbus.lvclass">)  [unwired: 7 in]
            n155 = call <vilib>:"BroadcastConnectionStatus.vi"("error in (no error)"=w499, "status"=ConnectionStatus."Offline", "Qbus in"=w498) -> ("error out"=w496:errorcluster)  [unwired: 7 in, 1 out]
            n156 = call <vilib>:"CloseConnectionInternal.vi"("error in (no error)"=w496, "Qbus in"=w519, "connected"=w525, "tcp reference"=w529) -> ("error out"=w515:errorcluster)  [unwired: 7 in]
            n157 = call <vilib>:"OpenTcpMessageConnection.vi"("timeout (ms)"=w500, "error in (no error)"=w515, "Port"=w527, "Hostname"=w528, "ClientName"=w504) -> ("error out"=w526:errorcluster, "connection ID out"=w523:T2)  [unwired: 5 in]
            n158 = call <vilib>:"DeviceReplyTo.vi"("Device"=w504) -> ("ReplyTo"=w503:string)  [unwired: 10 in]
            n159 = case shown="No Error" w526 {
              selector: w526 -> [w535 _]
              tunnel: w523 -> [w536 _]
              tunnel: [ConnectionStatus."NotAuthorized" ("status") ConnectionStatus."Offline" ("status")] -> w507
              tunnel: w521 -> [w538 _]
              tunnel: w504 -> [w537 _]
              tunnel: [w536 _] -> w520
              tunnel: [w534 w547] -> w512
              tunnel: [w531 w546] -> w518
              tunnel: [w533 _] -> w517
              tunnel: w515 -> [_ w547]
              tunnel: w503 -> [w532 _]
              tunnel: w500 -> [w530 _]
              frame No Error {
                n160 = To Variant(anything=w536) -> (Variant=w533:variant)
                n161 = call <vilib>:"Create Initiation Keys.vi"("error in"=w535, "srp"=w538) -> ("error out"=w543:errorcluster, "PUblicKeyA"=w542:u8[])  [unwired: 7 in, 1 out]
                n162 = Bundle By Name(cluster=T19 {"ClientName"="", "PublicKeyA"=[]} ("Body"), "ClientName"=w537, "PublicKeyA"=w542) -> (w541:T19)
                n163 = call <vilib>:"IntMsgSetTcpDvr.vi"() -> ("message name"=w531:string)  [unwired: 5 in]
                n164 = call <vilib>:"AuthSrpInitiationRequest_Create.vi"("error in (no error)"=w543, "AuthSrpInitiationRequest"=w541, "ReplyTo"=w532) -> ("error out"=w539:errorcluster, "Message"=w540:T21)  [unwired: 7 in]
                n165 = call <vilib>:"SendTcpMessage.vi"("timeout (5 sec)"=w530, "error in (no error)"=w539, "message"=w540, "connection ID in"=w536) -> ("error out"=w534:errorcluster)  [unwired: 5 in, 2 out]
              }
              frame Error {
                n166 = call <vilib>:"IntMsgClearTcpDvr.vi"() -> ("message name"=w546:string)  [unwired: 5 in]
              }
            }
            n167 = call <vilib>:"TcpReaderProcessName.vi"() -> ("process name"=w516:string)  [unwired: 5 in]
            n168 = call <vilib>:"SetConnectedStatus.vi"("status"=w507, "dvrConnected"=w525) -> ()  [unwired: 5 in, 1 out]
            n169 = call <vilib>:"SendRoutedMessage.vi"("listener process"=w516, "error in (no error)"=w512, "message value"=w517, "message name"=w518, "Qbus in"=w519) -> ("error in (no error)"=w511:errorcluster, "Qbus out"=w514:refnum<class "Qbus.lvclass">)  [unwired: 5 in]
            n170 = call <vilib>:"ConfigAuthenticationTimeout.vi"("timer function"=TimerFunction."Start" ("Timer function"), "error in (no error)"=w511, "reconnect in"=w513, "Qbus in"=w514) -> ("error out"=w508:errorcluster, "reconnect out"=w510:T8, "Qbus out"=w509:refnum<class "Qbus.lvclass">)  [unwired: 5 in]
            n171 = Bundle By Name(cluster=w502, "DataSend"=T6 {"SendFileMode"=enum."File", "data"=variant, "InProgress"=FALSE}, "Reconnect"=w510, "tcp"=w520) -> (w522:T1)
            n172 = call <vilib>:"BroadcastConnectionStatus.vi"("error in (no error)"=w508, "status"=w507, "Qbus in"=w509) -> ("error out"=w506:errorcluster)  [unwired: 7 in, 1 out]
          }
          frame True {
          }
        }
      }
      frame "ServerComm.CloseConnection" {
        n173 = Unbundle By Name(w559) -> ("tcp"=w564:T2, "connected"=w563:T5)
        n174 = call <vilib>:"TraceProvisioning.vi"("error in (no error)"=w562, "message name"=w560, "Qbus in"=w557) -> ("error out"=w561:errorcluster)  [unwired: 7 in, 1 out]
        n175 = call <vilib>:"CloseConnectionInternal.vi"("error in (no error)"=w561, "Qbus in"=w557, "connected"=w563, "tcp reference"=w564) -> ("error out"=w555:errorcluster)  [unwired: 7 in]
        n176 = call <vilib>:"IntMsgClearTcpDvr.vi"() -> ("message name"=w551:string)  [unwired: 5 in]
        n177 = call <vilib>:"TcpReaderProcessName.vi"() -> ("process name"=w556:string)  [unwired: 5 in]
        n178 = call <vilib>:"SendRoutedMessage.vi"("listener process"=w556, "error in (no error)"=w555, "message name"=w551, "Qbus in"=w557) -> ("error in (no error)"=w553:errorcluster)  [unwired: 6 in, 1 out]
        n179 = Bundle By Name(cluster=w559, "tcp"=T2 refnum) -> (w558:T1)
      }
      frame "ServerComm.SetConnectionInfo" {
        n180 = call <vilib>:"ParseSetConnectionInfo.vi"("error in (no error)"=w575, "body"=w574) -> ("error out"=w573:errorcluster, "connection info"=w567:T3)  [unwired: 8 in]
        n181 = call <vilib>:"WriteConnInfo.vi"("error in (no error)"=w573, "connection info"=w567) -> ("error out"=w572:errorcluster)  [unwired: 9 in]
        n182 = call <vilib>:"SendOpenConnection.vi"("error in (no error)"=w572, "Qbus in"=w569) -> ("error out"=w568:errorcluster)  [unwired: 8 in, 1 out]
        n183 = Bundle By Name(cluster=w571, "ConnInfo"=w567) -> (w570:T1)
      }
      frame "ServerComm.SetReconnectInterval" {
        n184 = call <vilib>:"ParseSetReconnectInterval.vi"("error in (no error)"=w583, "body"=w581) -> ("error out"=w582:errorcluster, "reconnect interval"=w578:dbl)  [unwired: 8 in]
        n185 = Bundle By Name(cluster=w580, "Reconnect.ReconnectInterval"=w578, "Reconnect.BaseReconnectInterval"=w578) -> (w579:T1)
      }
      frame "ServerComm.SendMessage" {
        n186 = call <vilib>:"ParseMessage.vi"("error in (no error)"=w596, "Body"=w595) -> ("error out"=w591:errorcluster, "Message"=w586:T21)  [unwired: 8 in]
        n187 = Unbundle By Name(w594) -> ("connected"=w593:T5, "tcp"=w590:T2)
        n188 = Unbundle By Name(w586) -> ("Header.MessageName"=w585:string)
        n189 = call <vilib>:"GetConnectedStatus.vi"("dvr connected"=w593) -> ("status"=w592:T12)  [unwired: 5 in, 1 out]
        n190 = case shown="\"Online\"" w592 {
          tunnel: w591 -> [w605 w607]
          tunnel: w586 -> [w602 w609]
          tunnel: w590 -> [_ w610]
          tunnel: [w603 w606] -> w589
          tunnel: w588 -> [w604 _]
          frame Default {
            w598 = -386730  # DeviceNotAuthorized
            n191 = To Variant(anything=w602) -> (Variant=w600:variant)
            n192 = call <vilib>:"SetErrorOnVariant.vi"("error code"=w598, "body in"=w600) -> ("body out"=w599:variant)  [unwired: 9 in]
            n193 = call <vilib>:"SendMessageErrorName.vi"() -> ("message name"=w601:string)  [unwired: 5 in]
            n194 = call <vilib>:"SendBroadcastMessage.vi"("error in (no error)"=w605, "message value"=w599, "message name"=w601, "Qbus in"=w604) -> ("error in (no error)"=w603:errorcluster)  [unwired: 6 in, 1 out]
          }
          frame "Online" {
            n195 = call <vilib>:"SendMessageInternal.vi"("timeout (5 sec)"=5000, "error in (no error)"=w607, "message"=w609, "connection ID in"=w610) -> ("error out"=w606:errorcluster)  [unwired: 6 in, 1 out]
          }
        }
      }
      frame "ServerComm.DataEventSendData" {
        n196 = Unbundle By Name(w625) -> ("DataSend"=w618:T6, "connected"=w619:T5, "tcp"=w627:T2, "ConnInfo.ClientName"=w614:string)
        n197 = Unbundle By Name(w618) -> ("InProgress"=w623:bool)
        n198 = call <vilib>:"GetConnectedStatus.vi"("dvr connected"=w619) -> ("status"=w620:T12)  [unwired: 5 in, 1 out]
        n199 = Equal?(x=w620, y=ConnectionStatus."Online") -> (x = y?=w616:bool)
        n200 = Not(x=w623) -> (.not. x?=w622:bool)
        n201 = And(x=w622, y=w616) -> (x .and. y?=w617:bool)
        n202 = case shown="True" w617 {
          tunnel: w627 -> [_ w657]
          tunnel: [w638 w662] -> w626
          tunnel: w612 -> [w639 w661]
          tunnel: w614 -> [_ w642]
          tunnel: w625 -> [w637 w660]
          tunnel: [w637 w659] -> w624
          tunnel: w616 -> [w635 _]
          tunnel: w613 -> [w630 w658]
          tunnel: w612 -> [_ _]
          tunnel: w611 -> [w631 w646]
          frame False {
            w633 = -386729  # BusySendingData
            w634 = -386730  # DeviceNotAuthorized
            n203 = Select(t=w633, s=w635, f=w634) -> (s? t:f=w632:i32)
            n204 = call <vilib>:"SetErrorOnVariant.vi"("error code"=w632, "body in"=w631) -> ("body out"=w636:variant)  [unwired: 9 in]
            n205 = call <vilib>:"SendDataReferenceResponseName.vi"() -> ("message name"=w629:string)  [unwired: 5 in]
            n206 = call <vilib>:"SendBroadcastMessage.vi"("error in (no error)"=w630, "message value"=w636, "message name"=w629, "Qbus in"=w639) -> ("error in (no error)"=w638:errorcluster)  [unwired: 6 in, 1 out]
          }
          frame True {
            n207 = call <vilib>:"ParseDataStorageSendData.vi"("error in (no error)"=w658, "body"=w646) -> ("error out"=w656:errorcluster, "DataEvent.Id"=w643:string)  [unwired: 4 in, 4 out]
            n208 = call <vilib>:"DeviceReplyTo.vi"("Device"=w642) -> ("ReplyTo"=w641:string)  [unwired: 10 in]
            n209 = call <vilib>:"SetCorrelationId.vi"("error in (no error)"=w656) -> ("error out"=w648:errorcluster, "correlation Id"=w645:string, "header out"=w640:T22)  [unwired: 8 in]
            n210 = Set Variant Attribute(Variant=w646, name="CorrId", value=w645, error in=w648) -> (Variant out=w644:variant, error out=w647:errorcluster)  [unwired: 1 out]
            n211 = Bundle By Name(cluster=T20 {"EventId"="", "Properties"=[]} ("DataStorageOpenEventRequest"), "EventId"=w643) -> (w652:T20)
            n212 = call <vilib>:"DataStorageOpenEventRequest_Create.vi"("Header"=w640, "error in (no error)"=w647, "DataStorageOpenEventRequest"=w652, "ReplyTo"=w641) -> ("error out"=w654:errorcluster, "Message"=w653:T21)  [unwired: 6 in]
            n213 = call <vilib>:"SendTcpMessage.vi"("timeout (5 sec)"=5000, "error in (no error)"=w654, "message"=w653, "connection ID in"=w657) -> ("error out"=w663:errorcluster)  [unwired: 5 in, 2 out]
            n214 = Bundle By Name(cluster=w660, "DataSend.SendFileMode"=DataSendMode."ByteArray", "DataSend.data"=w644, "DataSend.InProgress"=TRUE) -> (w659:T1)
            n215 = call <vilib>:"ConfigDataSendTimeout.vi"("error in (no error)"=w663, "Qbus in"=w661) -> ("error out"=w662:errorcluster)  [unwired: 8 in, 1 out]
          }
        }
      }
      frame "ServerComm.UpdatePassword" {
        n216 = call <vilib>:"ParseUpdatePassword.vi"("error in (no error)"=w668, "body"=w669) -> ("error out"=w667:errorcluster, "Update Password"=w665:T41)  [unwired: 8 in]
        n217 = call <vilib>:"SendEncryptedEndpointAuth.vi"("error in (no error)"=w667, "Update Password"=w665, "config"=w666) -> ("error out"=w670:errorcluster)  [unwired: 8 in]
      }
      frame "Start" {
        n218 = call <vilib>:"ReadConnInfo.vi"("error in (no error)"=w688) -> ("error out"=w682:errorcluster, "found"=w687:bool, "connection info"=w679:T3)  [unwired: 8 in]
        n219 = call <vilib>:"GetDevice.vi"("error in (no error)"=w682) -> ("error out"=w681:errorcluster, "device configuration"=w686:T42)  [unwired: 8 in, 1 out]
        n220 = Unbundle By Name(w686) -> ("ConfigurationVersion"=w684:string)
        n221 = case shown="True" w687 {
          tunnel: w680 -> [_ w695]
          tunnel: w681 -> [w692 w694]
          tunnel: [w692 w693] -> w678
          frame False {
          }
          frame True {
            n222 = call <vilib>:"SendOpenConnection.vi"("error in (no error)"=w694, "Qbus in"=w695) -> ("error out"=w693:errorcluster)  [unwired: 8 in, 1 out]
          }
        }
        n223 = call <vilib>:"GetMap.vi"() -> ("SystemInfoMap"=w676:T45)  [unwired: 10 in, 1 out]
        n224 = call <vilib>:"UpdateSystemInfoToMap.vi"("map in"=w676) -> ("system info"=w675:T46)  [unwired: 6 in, 4 out]
        n225 = Unbundle By Name(w675) -> ("ID"=w674:string, "Version"=w673:string)
        n226 = Bundle By Name(cluster=T9 {"ConfigurationVersion"="", "ApplicationVersion"="", "ApplicationType"=""} ("VersionInfo"), "ConfigurationVersion"=w684, "ApplicationType"=w674, "ApplicationVersion"=w673) -> (w683:T9)
        n227 = Bundle By Name(cluster=w690, "ConnInfo"=w679, "ProvVersionInfo"=w683) -> (w689:T1)
      }
      frame "Stop" {
        n228 = call <vilib>:"SendCloseConnection.vi"("error in (no error)"=w697, "Qbus in"=w696) -> ("error out"=w698:errorcluster)  [unwired: 8 in, 1 out]
      }
      frame "Exit" {
        n229 = Unbundle By Name(w712) -> ("SRP"=w705:T4, "tcp"=w711:T2, "connected"=w706:T5)
        n230 = call <vilib>:"CloseConnectionInternal.vi"("error in (no error)"=w702, "Qbus in"=w703, "connected"=w706, "tcp reference"=w711) -> ("error out"=w710:errorcluster)  [unwired: 7 in]
        n231 = flat-sequence {
          tunnel: w710 -> [_]
          tunnel: [w714] -> w708
          tunnel: [w715] -> w707
          tunnel: w706 -> [w717]
          tunnel: w705 -> [w716]
          frame #0 {
            n232 = call <vilib>:"Finalize.vi"("srp"=w716) -> ("error out"=w715:errorcluster)  [unwired: 10 in]
            n233 = Delete Data Value Reference(data value reference=w717) -> (error out=w714:errorcluster)  [unwired: 1 in, 1 out]
          }
        }
        n234 = Merge Errors(w707, w708, w710) -> (w709:errorcluster)
      }
    }
    n235 = Empty String/Path?(string/path=w45) -> (empty?=w46:bool)
    n236 = Select(t=w44, s=w46, f=w45) -> (s? t:f=w36:string)
    n237 = call <vilib>:"LoopState.vi"("error in (no error)"=w54, "loop action"=w36, "process name"=w42, "Qbus in"=w38) -> ("error out"=w53:errorcluster, "Qbus out"=w52:refnum<class "Qbus.lvclass">)  [unwired: 6 in]
    n238 = feedback #1() -> (w40:i32)  [unwired: 1 in]
    n239 = call <vilib>:"TcpErrorHandler.vi"("error in (no error)"=w53, "consequtive error count in"=w40, "Qbus in"=w52) -> ("error out"=w59:errorcluster, "consequtive error count out"=w41:i32, "Qbus out"=w57:refnum<class "Qbus.lvclass">)  [unwired: 6 in]
    n240 = feedback-in #1(w41) -> ()
    n241 = call <vilib>:"CatchError.vi"("source"=w42, "error in (no error)"=w59, "next action in"=w39, "Qbus in"=w57) -> ("error out"=w58:errorcluster, "next action out"=w55:string, "Qbus out"=w56:refnum<class "Qbus.lvclass">)  [unwired: 5 in]
  }
  n242 = call <vilib>:"TcpReaderProcess.vi"("error in (no error)"="error in (no error)", "Pound"="Pound in", "Qbus in"="Qbus in") -> ("error out"=w17:errorcluster)  [unwired: 8 in]
  n243 = call <vilib>:"TcpSendData.vi"("error in (no error)"="error in (no error)", "Pound in"="Pound in", "Qbus in"="Qbus in") -> ("error out"=w16:errorcluster)  [unwired: 8 in]
  n244 = call <vilib>:"Process.vi"("error in (no error)"="error in (no error)", "pound in"="Pound in", "qbus in"="Qbus in") -> ("error out"=w13:errorcluster)  [unwired: 8 in]
  n245 = call <vilib>:"Process.vi"("Pound in"="Pound in", "Qbus in"="Qbus in") -> ("error out"=w10:errorcluster)  [unwired: 9 in]
  n246 = Merge Errors(w17, w16, w13, w10) -> (w15:errorcluster)
  n247 = call <vilib>:"ShutdownMode.vi"("error in (no error)"=w23, "Watchdog"=w26) -> ("error out"=w25:errorcluster, "Watchdog"=w27:refnum<data-value>)  [unwired: 8 in]
  n248 = call <vilib>:"DestroyListenerProcess.vi"("error in (no error)"=w33, "process name"=w31, "Qbus in"=w32) -> ("error in (no error)"=w22:errorcluster)  [unwired: 7 in, 1 out]
  n249 = call <vilib>:"Close.vi"("error in (no error)"=w25, "Watchdog"=w27) -> ("error out"=w21:errorcluster)  [unwired: 9 in]
  n250 = Merge Errors(w21, w22, w15) -> (→"error out":errorcluster)
